vi "Read configuration.vi"(8 "error in":errorcluster, 11 "CVT Engine Editor in":refnum<class "CVT Engine Editor.lvclass">) -> (0 "error out":errorcluster, 2 "configuration":refnum<class "NISE_CEF_serializable configuration.lvclass">, 3 "CVT Engine Editor out":refnum<class "CVT Engine Editor.lvclass">)   [LabVIEW 2013, in "CVT Engine Editor.lvclass"]
uses:
  CVT Engine Editor.lvclass
  <vilib>/NI/Configuration Framework/serializable configuration/NISE_CEF_serializable configuration.lvclass
  CVT Engine Editor.lvclass/CVT Engine Editor.ctl
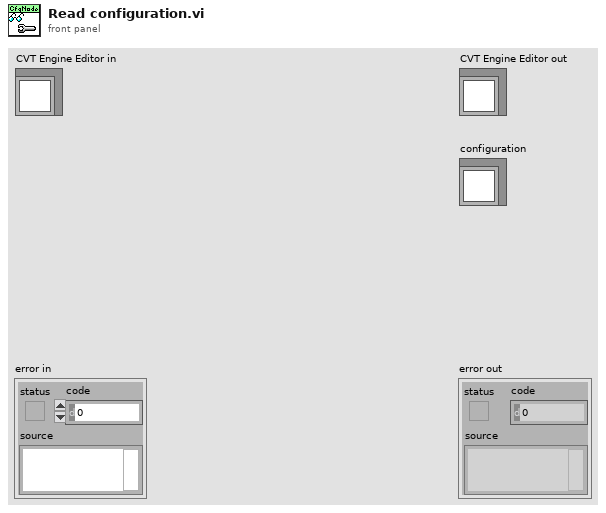
[diagram p1: front panel]
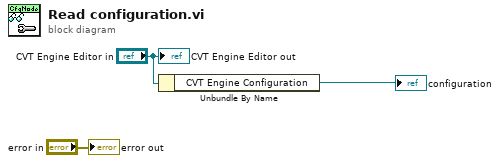
[diagram p0: block diagram]
diagram:
  n1 = Unbundle By Name("CVT Engine Editor in") -> ("CVT Engine Configuration"=→"configuration":refnum<class "CVT Engine Configuration.lvclass">)
  "error out" <- "error in"
  "CVT Engine Editor out" <- "CVT Engine Editor in"
